vi "File.vi"   [LabVIEW 2017]
types:
  T1 = enum16{"open", "replace", "create", "open or create", "replace or create", "replace or create with confirmation"}
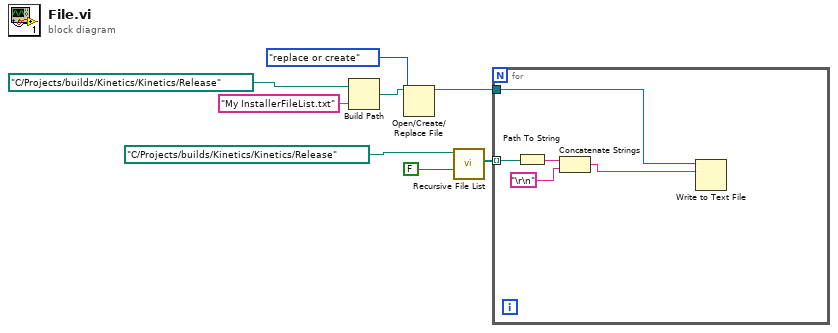
[diagram p0: block diagram]
diagram:
  n1 = Build Path(base path=path "C:/Projects/builds/Kinetics/Kinetics/Release", name or relative path="My InstallerFileList.txt") -> (appended path=w5:path)
  n2 = Open/Create/Replace File(file path (use dialog)=w5, operation (0:open)=T1."replace or create") -> (refnum out=w2:refnum<file>)  [unwired: 4 in, 2 out]
  n3 = call <vilib>:"Recursive File List.vi"("Continue Recursing on Error? (F)"=FALSE, "Folder Path"=path "C:/Projects/builds/Kinetics/Kinetics/Release") -> ("All Files in Dir"=w6:path[])  [unwired: 5 in, 4 out]
  n4 = for {
    tunnel: w6 -> [w13] mode=indexing
    tunnel: w2 -> [w11]
    n5 = Path To String(path=w13) -> (string=w12:string)
    n6 = Concatenate Strings(w12, "\r\n") -> (w10:string)
    n7 = Write to Text File(file (use dialog)=w11, text=w10) -> ()  [unwired: 2 in, 3 out]
  }
